vi "GetAvgGraph.vi"(9 "HV?":bool, 10 "HVGrph_In":waveform(dbl), 11 "Grph_In":waveform(dbl)[](array[waveform])) -> (2 "Numeric":i32, 3 "Grph_Avg":waveform(dbl))   [LabVIEW 2013]
uses:
  <vilib>/Analysis/baseanly.llb/Mean (DBL).vi
  <vilib>/Waveform/WDTOps.llb/WDT Get Waveform Time Array DBL.vi
  <vilib>/Analysis/NI_AALBase.lvlib
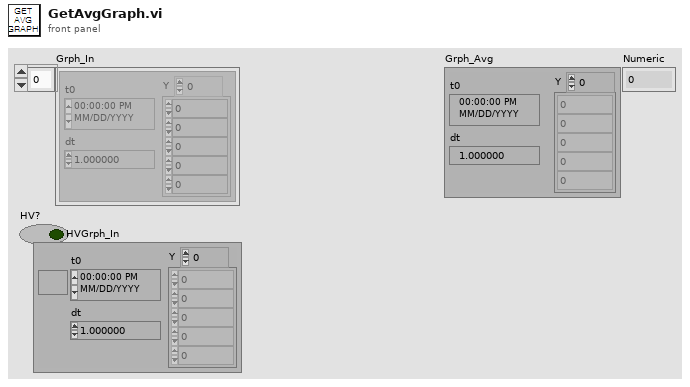
[diagram p1: front panel]
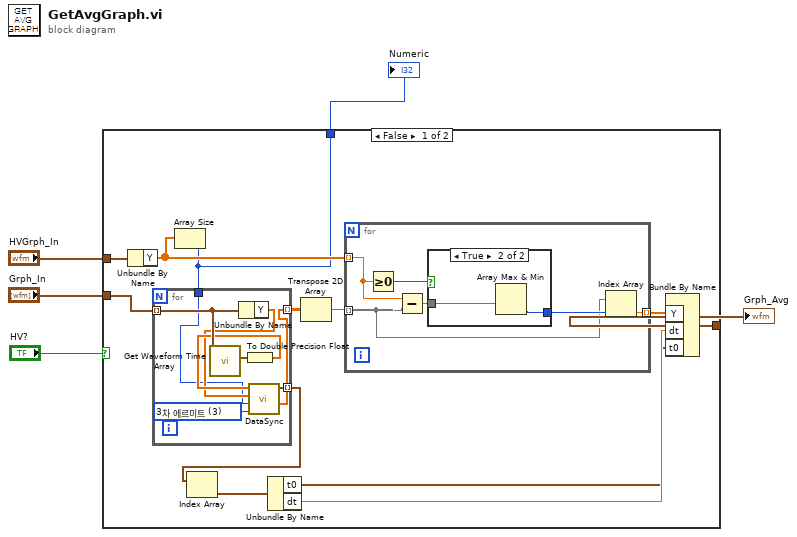
[diagram p0: block diagram]
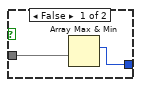
[diagram p2: hidden frame]
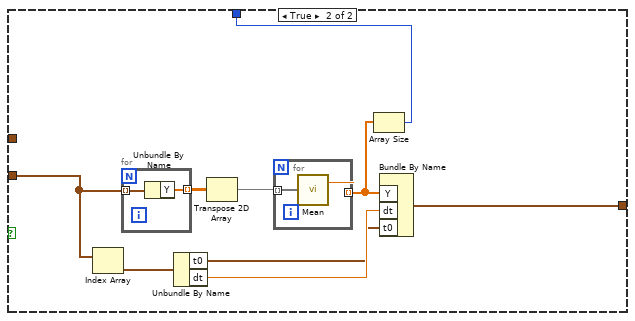
[diagram p3: hidden frame]
diagram:
  n1 = case shown="False" "HV?" {
    tunnel: "Grph_In" -> [w12 w39]
    tunnel: [w11 w38] -> w4
    tunnel: "HVGrph_In" -> [w10 _]
    tunnel: [w6 w36] -> w1
    frame False {
      n2 = Unbundle By Name(w10) -> ("Y"=w7:dbl[])
      n3 = Array Size(array=w7) -> (size(s)=w6:i32)
      n4 = for {
        tunnel: w12 -> [w35] mode=indexing
        tunnel: [w30] -> w17 mode=indexing
        tunnel: [w29] -> w8 mode=indexing
        tunnel: w6 -> [w28]
        w31 = 3 items=["최근접", "선형", "스플라인", "3차 에르미트", "라그랑지"] ("method")
        n5 = call-poly <vilib>:"Get Waveform Time Array.vi"("waveform in"=w35) -> ("X array"=w34:timestamp[])  [unwired: 9 in, 1 out]
        n6 = Unbundle By Name(w35) -> ("Y"=w32:dbl[])
        n7 = To Double Precision Float(number=w34) -> (double precision float=w33:dbl[])
        n8 = call "DataSync.vi"("method"=w31, "samples"=w28, "Y"=w32, "X"=w33) -> ("yi"=w30:dbl[], "출력 웨이브폼"=w29:waveform(dbl))  [unwired: 5 in, 1 out]
      }
      n9 = Index Array(array=w8) -> (element=w15:waveform(dbl))  [unwired: 1 in]
      n10 = Unbundle By Name(w15) -> ("t0"=w13:timestamp, "dt"=w14:dbl)
      n11 = Transpose 2D Array(2D array=w17) -> (transposed array=w9:dbl[][])
      n12 = for {
        tunnel: w9 -> [w19] mode=indexing
        tunnel: [w23] -> w16 mode=indexing
        tunnel: w7 -> [w20] mode=indexing
        n13 = Greater Or Equal To 0?(x=w20) -> (x >= 0?=w21:bool)
        n14 = Subtract(x=w20, y=w19) -> (x-y=w18:dbl[])
        n15 = case shown="True" w21 {
          tunnel: [w25 w27] -> w22
          tunnel: w18 -> [w24 w26]
          frame False {
            n16 = Array Max & Min(array=w24) -> (max index (indices)=w25:i32)  [unwired: 3 out]
          }
          frame True {
            n17 = Array Max & Min(array=w26) -> (min index (indices)=w27:i32)  [unwired: 3 out]
          }
        }
        n18 = Index Array(array=w19, index=w22) -> (element=w23:dbl)
      }
      n19 = Bundle By Name("Y"=w16, "dt"=w14, "t0"=w13) -> (w11:waveform(dbl))  [unwired: 1 in]
    }
    frame True {
      n20 = Index Array(array=w39) -> (element=w42:waveform(dbl))  [unwired: 1 in]
      n21 = for {
        tunnel: w39 -> [w48] mode=indexing
        tunnel: [w47] -> w44 mode=indexing
        n22 = Unbundle By Name(w48) -> ("Y"=w47:dbl[])
      }
      n23 = Unbundle By Name(w42) -> ("t0"=w40:timestamp, "dt"=w41:dbl)
      n24 = Transpose 2D Array(2D array=w44) -> (transposed array=w43:dbl[][])
      n25 = for {
        tunnel: w43 -> [w46] mode=indexing
        tunnel: [w45] -> w37 mode=indexing
        n26 = call-poly <vilib>:"Mean.vi"("X"=w46) -> ("mean"=w45:dbl)  [unwired: 1 out]
      }
      n27 = Array Size(array=w37) -> (size(s)=w36:i32)
      n28 = Bundle By Name("Y"=w37, "dt"=w41, "t0"=w40) -> (w38:waveform(dbl))  [unwired: 1 in]
    }
  }
  "Grph_Avg" <- w4
  "Numeric" <- w1
